vi "IAmGLF-CreateDVR.vi"(8 "error in (no error)":errorcluster, 11 "Engine in":refnum<class "Engine.lvclass">) -> (0 "error out":errorcluster, 3 "Engine out":refnum<class "Engine.lvclass">)   [LabVIEW 2024, in "GLF.lvlib" / "Engine.lvclass"]
doc: "<B>Summary</B>\nTo create the class DVR in an standalone process."
uses:
  Engine.lvclass
  Engine.lvclass/Engine.ctl
  DVR--cluster.ctl
  Metrics--cluster.ctl
  Context--cluster.ctl
  Config--cluster.ctl
  VSync--enum.ctl
  Command--queue.ctl
  Command--cluster.ctl
  Command--enum.ctl
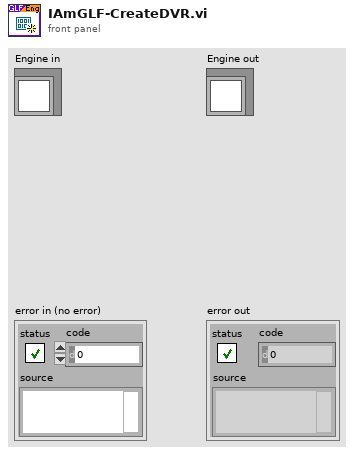
[diagram p1: front panel]
types:
  T1 = typedef "GLF.lvlib/Engine.lvclass/DVR--cluster.ctl" = cluster{"CMD Queue":T2, "Config":T3, "Ctxt":T5, "Metrics":T6}
  T2 = typedef "GLF.lvlib/Engine.lvclass/Command--queue.ctl" = refnum<queue>
  T3 = typedef "GLF.lvlib/Engine.lvclass/Config--cluster.ctl" = cluster{"Quit On Last Window Closed":bool, "VSync":T4, "FPS Target":dbl}
  T4 = typedef "GLF.lvlib/Engine.lvclass/VSync--enum.ctl" = enum16{"Disabled", "Enabled", "Adaptative"}
  T5 = typedef "GLF.lvlib/Engine.lvclass/Context--cluster.ctl" = cluster{"Ticks Begin":u64, "VSync Enabled":bool}
  T6 = typedef "GLF.lvlib/Engine.lvclass/Metrics--cluster.ctl" = cluster{"Uptime [ms]":u64, "Loop Time [ms]":u64}
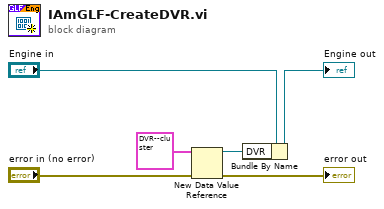
[diagram p0: block diagram]
diagram:
  n1 = New Data Value Reference(data value=T1 {"CMD Queue"=refnum, "Config"={"Quit On Last Window Closed"=FALSE, "VSync"=enum."Disabled", "FPS Target"=0.0}, "Ctxt"={"Ticks Begin"=0, "VSync Enabled"=FALSE}, "Metrics"={"Uptime [ms]"=0, "Loop Time [ms]"=0}} ("DVR"), error in="error in (no error)") -> (data value reference=w6:refnum<data-value>, error out=→"error out":errorcluster)
  n2 = Bundle By Name(cluster="Engine in", "DVR"=w6) -> (→"Engine out":refnum<class "Engine.lvclass">)
